vi "FindBall.vi"(8 "error out":errorcluster, 10 "Ball Color":T4, 11 "Data Highway Out":T2={"New Image"=refnum, "Session Out"="", "LIDAR VISA Name"="", "Phidget Device Out"=0, "Lidar Data"=[], "polar attributes"={"maximum"=0.0, "minimum"=0.0, "clip to min"=FALSE, "log?(F)"=FALSE, "grid color"=6710886, "plot color"=65280, "fmt and prec"={"format"=enum."Decimal", "precision"=0}, "visible section"=8}, "Debug Message"="", "Servo Angles"={"Angle X"=0.0, "Angle Y"=0.0}, "ColorPlane"=refnum, "Threshold"=refnum, "PartFilt"=refnum, "Processed Image"=refnum, "Magnitude"=[], "Direction"=[]} {"polar attributes"."minimum" format="%0.2f"; "polar attributes"."maximum" format="%0.2f"}) -> (0 "error out 2":errorcluster, 1 "Ball 2":dbl[](array[numeric]), 2 "Ball 1":dbl[](array[numeric]), 3 "Data Highway Out 2":T2={"New Image"=refnum, "Session Out"="", "LIDAR VISA Name"="", "Phidget Device Out"=0, "Lidar Data"=[], "polar attributes"={"maximum"=0.0, "minimum"=0.0, "clip to min"=FALSE, "log?(F)"=FALSE, "grid color"=6710886, "plot color"=65280, "fmt and prec"={"format"=enum."Decimal", "precision"=0}, "visible section"=8}, "Debug Message"="", "Servo Angles"={"Angle X"=0.0, "Angle Y"=0.0}, "ColorPlane"=refnum, "Threshold"=refnum, "PartFilt"=refnum, "Processed Image"=refnum, "Magnitude"=[], "Direction"=[]} {"polar attributes"."minimum" format="%0.2f"; "polar attributes"."maximum" format="%0.2f"})   [LabVIEW 2014]
uses:
  controls/Data.ctl
  <vilib>/vision/Image Controls.llb/IMAQ Image.ctl
  <vilib>/userdefined/High Color/IMAQdx.ctl
  controls/BallColor.ctl
  <vilib>/vision/NI_Vision_Development_Module.lvlib
panel:
  out "Processed Image":T1(plugin-control)
  out "Raw Image":T1(plugin-control)
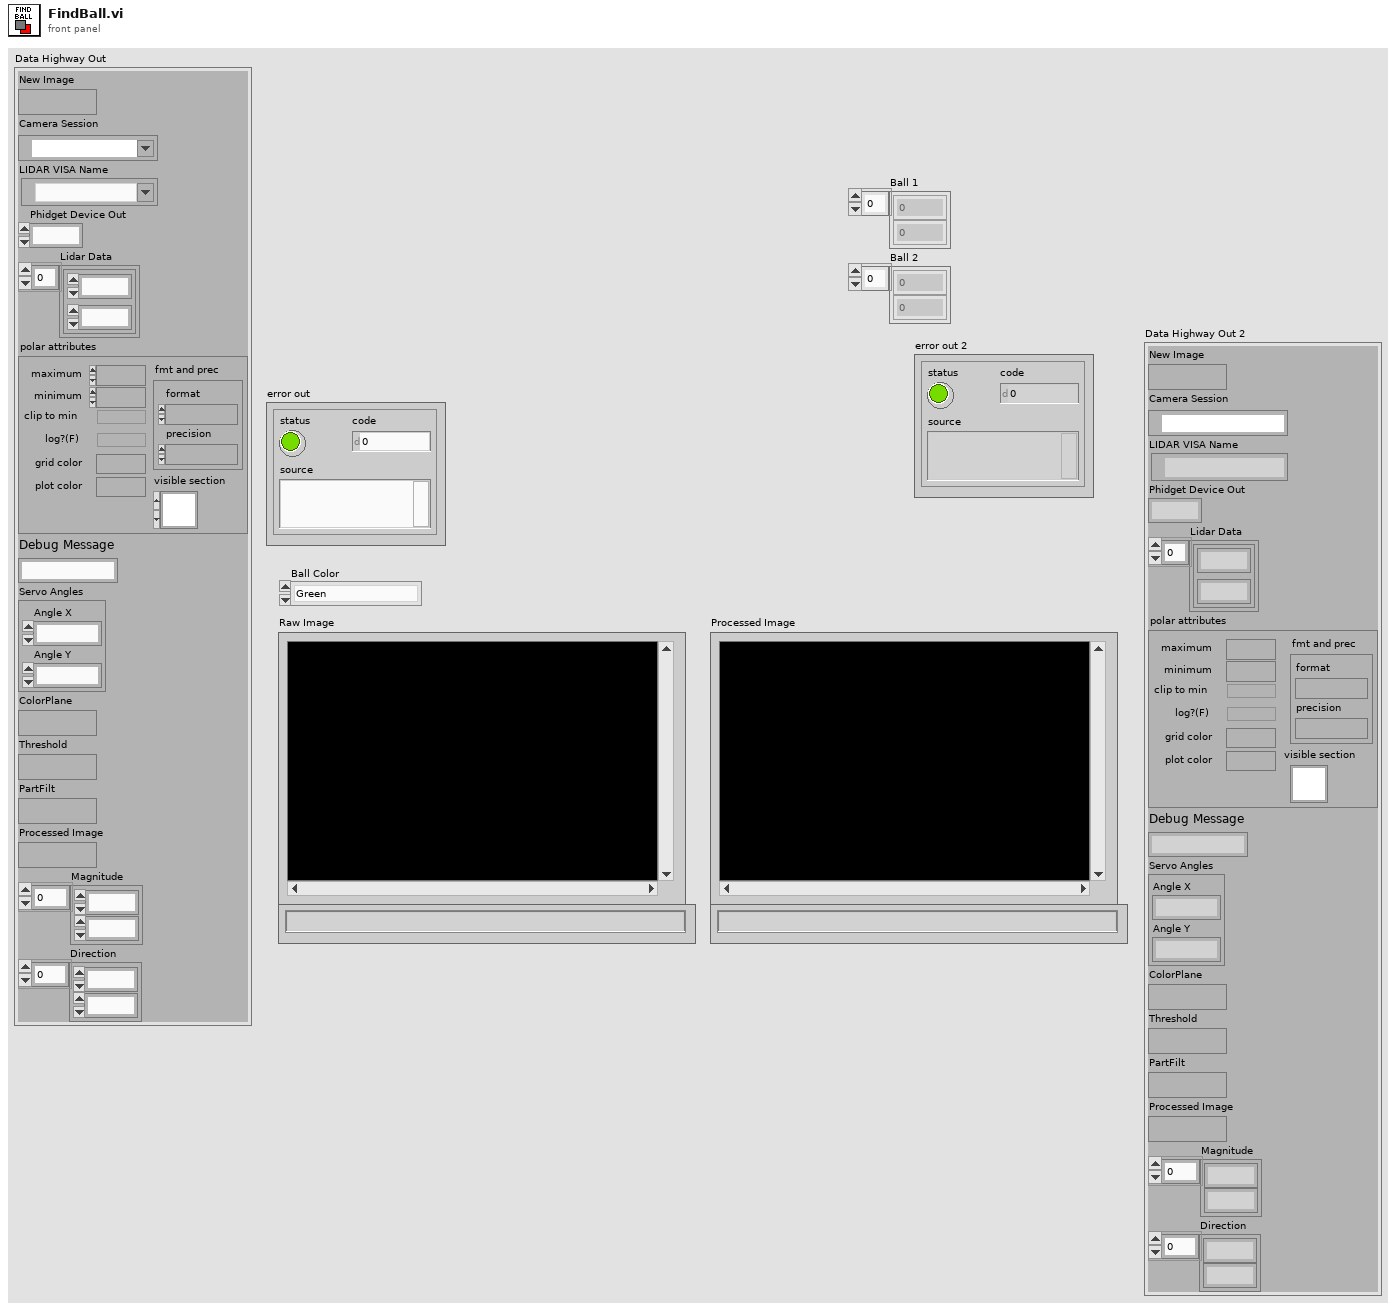
[diagram p1: front panel]
types:
  T1 = typedef "IMAQ Image.ctl" = refnum<image>
  T2 = typedef "Data.ctl" = cluster{"New Image":T1, "Session Out":T3, "LIDAR VISA Name":refnum<visa-resource-name>, "Phidget Device Out":i32, "Lidar Data":cluster{dbl, dbl}[], "polar attributes":cluster{"maximum":dbl, "minimum":dbl, "clip to min":bool, "log?(F)":bool, "grid color":u32, "plot color":u32, "fmt and prec":cluster{"format":enum8{"Decimal", "Scientific", "Engineering", "Binary", "Octal", "Hex"}, "precision":u8}, "visible section":u16}, "Debug Message":string, "Servo Angles":cluster{"Angle X":dbl, "Angle Y":dbl}, "ColorPlane":T1, "Threshold":T1, "PartFilt":T1, "Processed Image":T1, "Magnitude":dbl[], "Direction":dbl[]}
  T3 = typedef "IMAQdx.ctl" = refnum<k21>
  T4 = typedef "BallColor.ctl" = enum16{"Green", "Red"}
  T5 = typedef "Particle Parameters" = i32
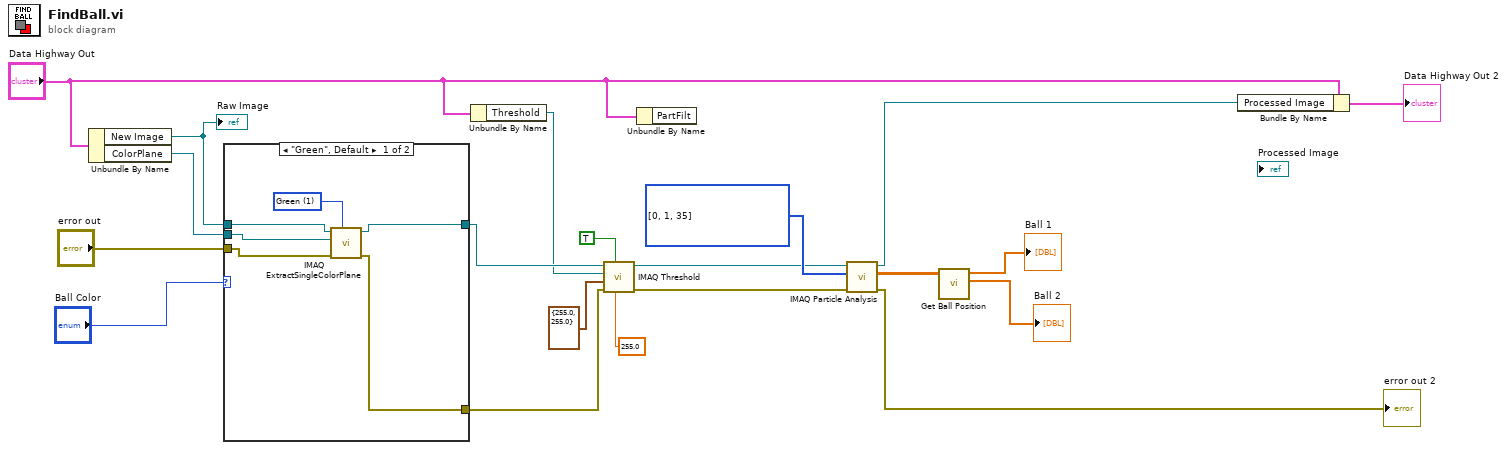
[diagram p0: block diagram]
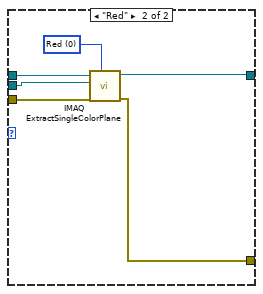
[diagram p2: hidden frame]
diagram:
  w8 = T5[] [0, 1, 35] items=["Center of Mass X", "Center of Mass Y", "First Pixel X", "First Pixel Y", "Bounding Rect Left", "Bounding Rect Top", "Bounding Rect Right", "Bounding Rect Bottom", "Max Feret Diameter Start X", "Max Feret Diameter Start Y", "Max Feret Diameter End X", "Max Feret Diameter End Y", "Max Horiz. Segment Length Left", "Max Horiz. Segment Length Right", "Max Horiz. Segment Length Row", "-", "Bounding Rect Width", "Bounding Rect Height", "Bounding Rect Diagonal", "Perimeter", "Convex Hull Perimeter", "Holes' Perimeter", "Max Feret Diameter", "Equivalent Ellipse Major Axis", "Equivalent Ellipse Minor Axis", "Equivalent Ellipse Minor Axis (Feret)", "Equivalent Rect Long Side", "Equivalent Rect Short Side", "Equivalent Rect Diagonal", "Equivalent Rect Short Side (Feret)", "Average Horiz. Segment Length", "Average Vert. Segment Length", "Hydraulic Radius", "Waddel Disk Diameter", "-", "Area", "Holes' Area", "Particle & Holes' Area", "Convex Hull Area", "Image Area", "-", "Number of Holes", "Number of Horiz. Segments", "Number of Vert. Segments", "-", "Orientation", "Max Feret Diameter Orientation", "-", "% Area/Image Area", "% Area/(Particle & Holes' Area)", "Ratio of Equivalent Ellipse Axes", "Ratio of Equivalent Rect Sides", "-", "Elongation Factor", "Compactness Factor", "Heywood Circularity Factor", "Type Factor", "-", "Sum X", "Sum Y", "Sum XX", "Sum XY", "Sum YY", "Sum XXX", "Sum XXY", "Sum XYY", "Sum YYY", "-", "Moment of Inertia XX", "Moment of Inertia XY", "Moment of Inertia YY", "Moment of Inertia XXX", "Moment of Inertia XXY", "Moment of Inertia XYY", "Moment of Inertia YYY", "Norm. Moment of Inertia XX", "Norm. Moment of Inertia XY", "Norm. Moment of Inertia YY", "Norm. Moment of Inertia XXX", "Norm. Moment of Inertia XXY", "Norm. Moment of Inertia XYY", "Norm. Moment of Inertia YYY", "Hu Moment 1", "Hu Moment 2", "Hu Moment 3", "Hu Moment 4", "Hu Moment 5", "Hu Moment 6", "Hu Moment 7"] ("Pixel Measurements")
  n1 = Unbundle By Name("Data Highway Out") -> ("New Image"=w17:T1, "ColorPlane"=w16:T1)
  "Raw Image" <- w17
  n2 = case shown="\"Green\", Default" "Ball Color" {
    tunnel: "error out" -> [w23 w29]
    tunnel: [w22 w31] -> w15
    tunnel: w17 -> [w25 w32]
    tunnel: [w21 w28] -> w13
    tunnel: w16 -> [w24 w30]
    frame "Green", Default {
      w26 = 1 items=["Red", "Green", "Blue", "Hue", "Saturation", "Luminance", "Value", "Intensity"] ("Color Plane")
      n3 = call "IMAQ ExtractSingleColorPlane"("Color Plane"=w26, "error in (no error)"=w23, "Image Dst"=w24, "Image Src"=w25) -> ("error out"=w21:errorcluster, "Image Dst Out"=w22:T1)  [unwired: 6 in]
    }
    frame "Red" {
      w27 = 0 items=["Red", "Green", "Blue", "Hue", "Saturation", "Luminance", "Value", "Intensity"] ("Color Plane")
      n4 = call "IMAQ ExtractSingleColorPlane"("Color Plane"=w27, "error in (no error)"=w29, "Image Dst"=w30, "Image Src"=w32) -> ("error out"=w28:errorcluster, "Image Dst Out"=w31:T1)  [unwired: 6 in]
    }
  }
  n5 = Unbundle By Name("Data Highway Out") -> ("Threshold"=w12:T1)
  n6 = call "IMAQ Threshold"("Replace Value"=sgl 255.0, "Keep/Replace Value (Replace)"=TRUE, "error in (no error)"=w13, "Range"=cluster{"Lower value":sgl, "Upper value":sgl} {"Lower value"=255.0, "Upper value"=255.0}, "Image Dst"=w12, "Image Src"=w15) -> ("error out"=w7:errorcluster, "Image Dst Out"=w2:T1)  [unwired: 4 in]
  n7 = Unbundle By Name("Data Highway Out") -> ()  [unwired: 1 out]
  n8 = call "IMAQ Particle Analysis"("error in (no error)"=w7, "Pixel Measurements"=w8, "Image"=w2) -> ("error out"=→"error out 2":errorcluster, "Particle Measurements (Pixels)"=w5:dbl[][], "Image Out (duplicate)"=w1:T1)  [unwired: 3 in, 3 out]
  n9 = call "Get Ball Position.vi"("Particle Measurements (Pixels)"=w5) -> ("Ball 2"=→"Ball 2":dbl[], "Ball 1"=→"Ball 1":dbl[])  [unwired: 9 in]
  n10 = Bundle By Name(cluster="Data Highway Out", "Processed Image"=w1) -> (→"Data Highway Out 2":T2)
